vi "Write and Read Multiple Registers.vi"(4 "read count":u16, 6 "read starting address":u16, 8 "error in (no error)":errorcluster, 9 "write values":u16[](array[numeric]), 10 "write starting address":u16, 11 "device data model in":refnum<class "ICPCON ET Data Model.lvclass">) -> (0 "error out":errorcluster, 1 "read values":u16[](array[numeric]), 3 "device data model out":refnum<class "ICPCON ET Data Model.lvclass">)   [LabVIEW 2021, in "ICPCON ET Data Model.lvclass"]
doc: "Writes and reads the values of multiple register values in series. The <b>write values</b> are inserted starting at <b>write starting address</b> and the returned <b>read values</b> consists of <b>read count</b> holding registers starting at <b>read starting address</b>."
uses:
  ICPCON ET Data Model.lvclass
  ICPCON ET Data Model.lvclass/ICPCON ET Data Model.ctl
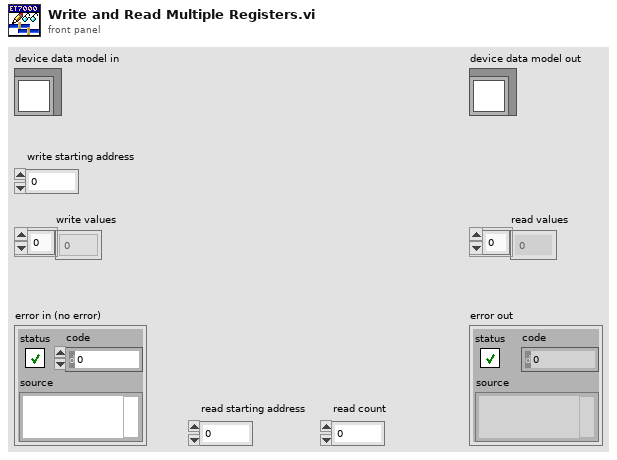
[diagram p1: front panel]
types:
  T1 = typedef "ICPCON ET Data Model.lvclass/Data Model.ctl" = cluster{"UTC":u64, "DI":bool[], "DO":bool[], "IR":u16[], "HR":u16[], "ES":u8}
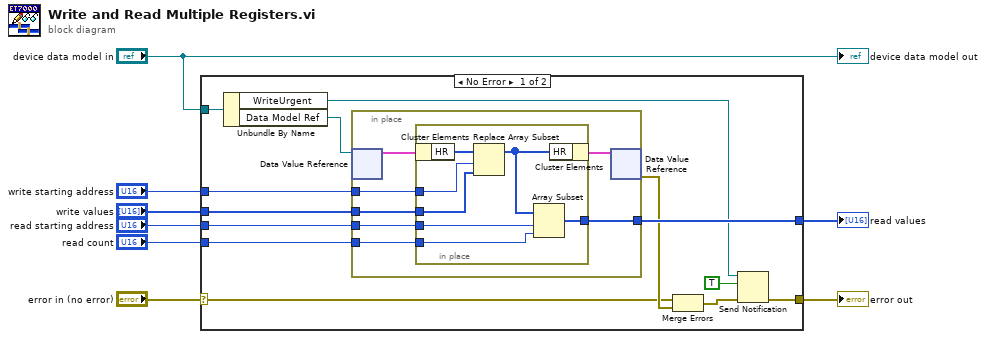
[diagram p0: block diagram]
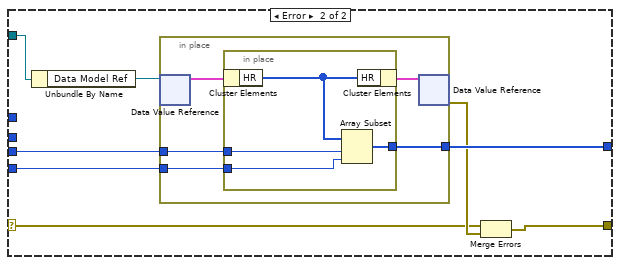
[diagram p2: hidden frame]
diagram:
  n1 = case shown="No Error" "error in (no error)" {
    selector: "error in (no error)" -> [w13 w36]
    tunnel: [w10 w43] -> w8
    tunnel: "write values" -> [w21 _]
    tunnel: "write starting address" -> [w20 _]
    tunnel: [w19 w42] -> w5
    tunnel: "read count" -> [w18 w41]
    tunnel: "read starting address" -> [w17 w40]
    tunnel: "device data model in" -> [w16 w39]
    frame No Error {
      n2 = Unbundle By Name(w16) -> ("WriteUrgent"=w9:refnum<notifier>, "Data Model Ref"=w15:refnum<data-value>)
      n3 = in-place {
        in-place-border: w21 -> [w28]
        in-place-border: w20 -> [w27]
        in-place-border: [w22] -> w19
        in-place-border: w18 -> [w23]
        in-place-border: w17 -> [w24]
        n4 = in-place-dvr #1(w15) -> (w26:T1)  [unwired: 1 out]
        n5 = in-place {
          in-place-border: w28 -> [w35]
          in-place-border: w27 -> [w34]
          in-place-border: w24 -> [w31]
          in-place-border: w23 -> [w30]
          in-place-border: [w29] -> w22
          n6 = in-place-cluster #2(w26) -> ("HR"=w33:u16[])
          n7 = Replace Array Subset(array=w33, new element=w35, index=w34) -> (w32:u16[])
          n8 = Array Subset(array=w32, index=w31, length=w30) -> (w29:u16[])
          n9 = in-place-cluster #2("HR"=w32) -> (w25:T1)
        }
        n10 = in-place-dvr #1(w25) -> (w14:errorcluster)  [unwired: 1 out]
      }
      n11 = Merge Errors(w13, w14) -> (w11:errorcluster)
      n12 = Send Notification(notification=TRUE, notifier=w9, error in (no error)=w11) -> (error out=w10:errorcluster)  [unwired: 1 out]
    }
    frame Error {
      n13 = Unbundle By Name(w39) -> ("Data Model Ref"=w38:refnum<data-value>)
      n14 = in-place {
        in-place-border: [w44] -> w42
        in-place-border: w41 -> [w45]
        in-place-border: w40 -> [w46]
        n15 = in-place-dvr #3(w38) -> (w48:T1)  [unwired: 1 out]
        n16 = in-place {
          in-place-border: w46 -> [w52]
          in-place-border: w45 -> [w51]
          in-place-border: [w50] -> w44
          n17 = in-place-cluster #4(w48) -> ("HR"=w49:u16[])
          n18 = Array Subset(array=w49, index=w52, length=w51) -> (w50:u16[])
          n19 = in-place-cluster #4("HR"=w49) -> (w47:T1)
        }
        n20 = in-place-dvr #3(w47) -> (w37:errorcluster)  [unwired: 1 out]
      }
      n21 = Merge Errors(w36, w37) -> (w43:errorcluster)
    }
  }
  "error out" <- w8
  "read values" <- w5
  "device data model out" <- "device data model in"
